vi "SVMDense_Train_FromFile.vi"() -> ()   [LabVIEW 2015]
uses:
  LibSVM Sparse/Controls/Kernel.ctl
  LibSVM Sparse/Wrapper API/Controls/svm_kernel_type.ctl
  LibSVM Sparse/Controls/Options Training.ctl
  LibSVM Sparse/Controls/Parameters NU_SVC.ctl
  Wrapper API/Controls/svmdense_model.ctl
  LibSVM Sparse/Wrapper API/Controls/svm_parameter.ctl
  LibSVM Sparse/Wrapper API/Controls/svm_type.ctl
  Tools/Controls/Binary_ConfusionMatrix.ctl
  SubVIs/SVM Dense Train NU_SVC.vi
  Tools/SubVIs/Dense - Scale Nodes Linear.vi
  Tools/SubVIs/Dense - Scale Problem Linear.vi
  Wrapper API/svmdense_train.vi
  Wrapper API/svmdense_predict.vi
panel:
  out "Binary Confusion Matrix":T1
  out "error out":errorcluster
  out "Model":T2
  in  "nu":T6=0.2 caption="nu (0,5)"
  in  "Options":T7={"cache_size"=500.0, "eps"=0.001, "shrinking"=TRUE, "probability"=FALSE}
  in  "Kernel":T8
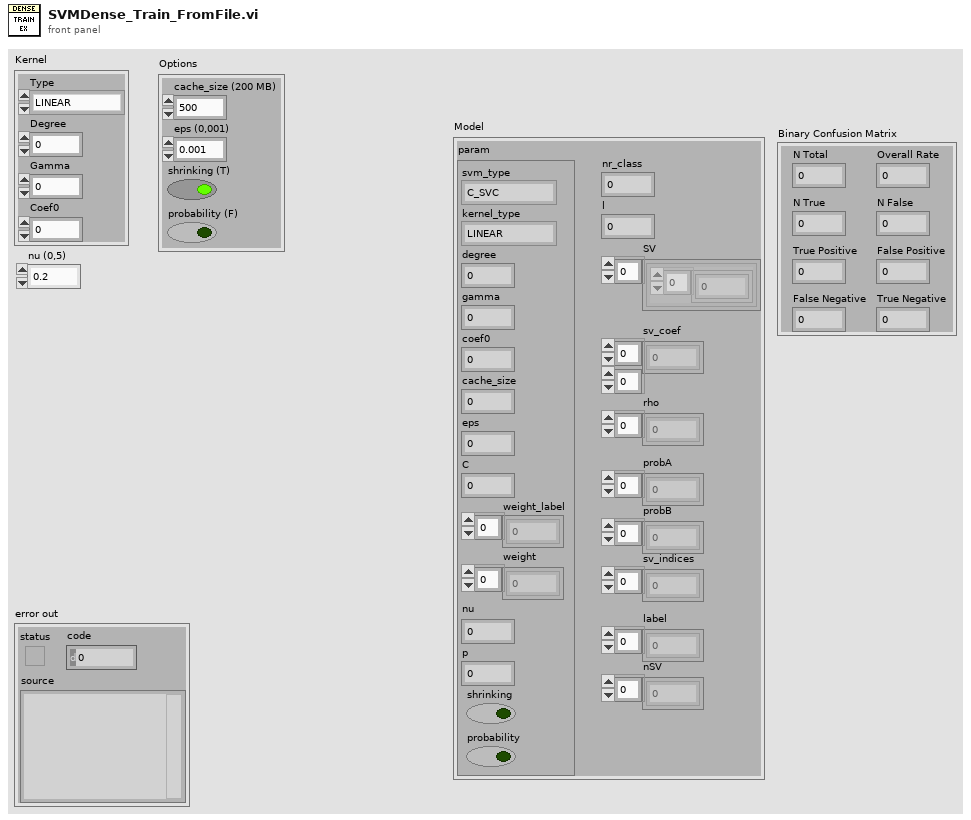
[diagram p1: front panel]
types:
  T1 = typedef "Binary_ConfusionMatrix.ctl" = cluster{"N Total":u32, "N True":u32, "N False":u32, "Overall Rate":dbl, "True Positive":dbl, "False Positive":dbl, "False Negative":dbl, "True Negative":dbl}
  T2 = typedef "svmdense_model.ctl" = cluster{"param":T3, "nr_class":i32, "l":i32, "SV":cluster{"Array":dbl[]}[], "sv_coef":dbl[][], "rho":dbl[], "probA":dbl[], "probB":dbl[], "sv_indices":i32[], "label":i32[], "nSV":i32[]}
  T3 = typedef "svm_parameter.ctl" = cluster{"svm_type":T4, "kernel_type":T5, "degree":i32, "gamma":dbl, "coef0":dbl, "cache_size":dbl, "eps":dbl, "C":dbl, "weight_label":i32[], "weight":dbl[], "nu":dbl, "p":dbl, "shrinking":bool, "probability":bool}
  T4 = typedef "svm_type.ctl" = enum32{"C_SVC", "NU_SVC", "ONE_CLASS", "EPSILON_SVR", "NU_SVR"}
  T5 = typedef "svm_kernel_type.ctl" = enum32{"LINEAR", "POLY", "RBF", "SIGMOID", "PRECOMPUTED"}
  T6 = typedef "Parameters NU_SVC.ctl" = dbl
  T7 = typedef "Options Training.ctl" = cluster{"cache_size":dbl, "eps":dbl, "shrinking":bool, "probability":bool}
  T8 = typedef "Kernel.ctl" = cluster{"Type":T5, "Degree":i32, "Gamma":dbl, "Coef0":dbl}
  T9 = typedef "svm_problem.ctl" = cluster{"y":dbl[], "x":cluster{T10[]}[]}
  T10 = typedef "svm_node.ctl" = cluster{"index":i32, "value":dbl}
  T11 = typedef "svmdense_problem.ctl" = cluster{"Y":dbl[], "X":cluster{"x":dbl[]}[]}
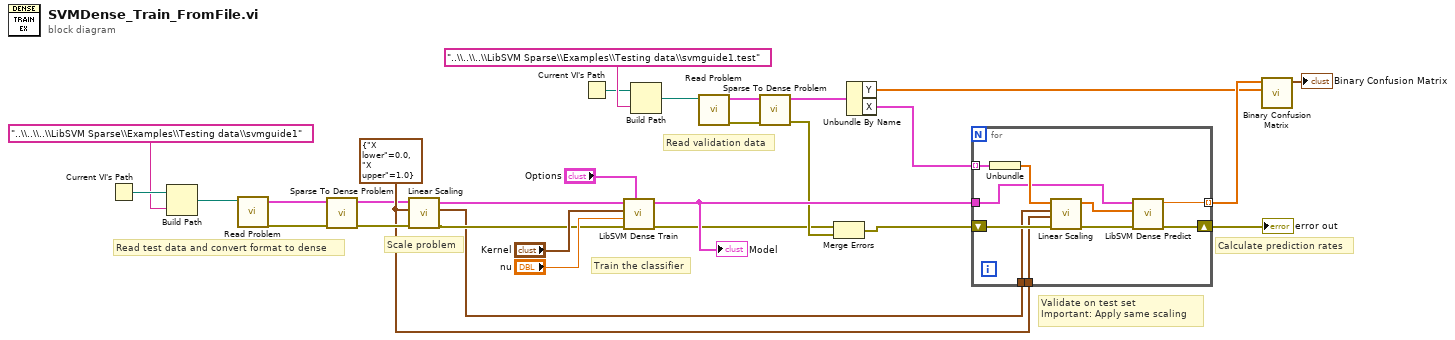
[diagram p0: block diagram]
diagram:
  w6 = cluster{"X lower":dbl, "X upper":dbl} {"X lower"=0.0, "X upper"=1.0} ("X Scaling limits")
  # "Calculate prediction rates"
  # "Scale problem"
  # "Read validation data"
  # "Read test data and convert format to dense"
  # "Train the classifier"
  # "Validate on test set\nImportant: Apply same scaling"
  n1 = Current VI's Path() -> (path=w28:path)
  n2 = Build Path(base path=w28, name or relative path="..\\..\\..\\LibSVM Sparse\\Examples\\Testing data\\svmguide1") -> (appended path=w29:path)
  n3 = call "Read Problem.vi"("file path (use dialog)"=w29) -> ("error out"=w23:errorcluster, "svm_problem"=w22:T9)  [unwired: 9 in]
  n4 = call "Sparse To Dense Problem.vi"("error in (no error)"=w23, "Sparse Problem"=w22) -> ("error out"=w10:errorcluster, "Dense Problem"=w2:T11)  [unwired: 8 in]
  n5 = call-poly "Linear Scaling.vi"("error in (no error)"=w10, "X Scaling limits"=w6, "Problem"=w2) -> ("error out"=w14:errorcluster, "xmaxmin"=w9:cluster{"min":dbl, "max":dbl}[], "Scaled problem"=w16:T11)  [unwired: 5 in, 1 out]
  n6 = Current VI's Path() -> (path=w26:path)
  n7 = call-poly "LibSVM Dense Train.vi"("Options"="Options", "error in (no error)"=w14, "nu"="nu", "Kernel"="Kernel", "Dense problem"=w16) -> ("error out"=w11:errorcluster, "Model"=w15:T2)  [unwired: 5 in]
  "Model" <- w15
  n8 = Build Path(base path=w26, name or relative path="..\\..\\..\\LibSVM Sparse\\Examples\\Testing data\\svmguide1.test") -> (appended path=w25:path)
  n9 = call "Read Problem.vi"("file path (use dialog)"=w25) -> ("error out"=w17:errorcluster, "svm_problem"=w24:T9)  [unwired: 9 in]
  n10 = call "Sparse To Dense Problem.vi"("error in (no error)"=w17, "Sparse Problem"=w24) -> ("error out"=w12:errorcluster, "Dense Problem"=w8:T11)  [unwired: 8 in]
  n11 = Merge Errors(w11, w12) -> (w13:errorcluster)
  n12 = Unbundle By Name(w8) -> ("Y"=w4:dbl[], "X"=w7:cluster{"x":dbl[]}[])
  n13 = for {
    tunnel: w15 -> [w31]
    shift-right: [w39] -> w1
    shift-left: w13 -> [w37]
    tunnel: [w38] -> w5 mode=indexing
    tunnel: w9 -> [w33]
    tunnel: w7 -> [w35] mode=indexing
    tunnel: w6 -> [w32]
    n14 = Unbundle(w35) -> ("x"=w34:dbl[])
    n15 = call-poly "Linear Scaling.vi"("error in (no error)"=w37, "Scaling limits"=w32, "xmaxmin"=w33, "x"=w34) -> ("error out"=w36:errorcluster, "x scaled"=w30:dbl[])  [unwired: 6 in]
    n16 = call-poly "LibSVM Dense Predict.vi"("error in (no error)"=w36, "x"=w30, "Model"=w31) -> ("error out"=w39:errorcluster, "Predicted label"=w38:dbl)  [unwired: 7 in]
  }
  "error out" <- w1
  n17 = call "Binary Confusion Matrix.vi"("Actual Labels"=w4, "Predicted Labels"=w5) -> ("Binary Confusion Matrix"=→"Binary Confusion Matrix":T1)  [unwired: 9 in]
